vi "Get SMO Port.vi"(8 "error in (no error)":errorcluster, 11 "Inst.FPInstrument in":refnum<class "Inst.FP.lvclass">) -> (0 "error out":errorcluster, 2 "Port":u16, 3 "Inst.FPInstrument out":refnum<class "Inst.FP.lvclass">)   [LabVIEW 2019, in "Inst.FP.lvclass"]
uses:
  Inst.FP.lvclass
  <userlib>/LevyLab/Instrument Framework/Instrument Types/VSource/Instrument.VSource.lvclass
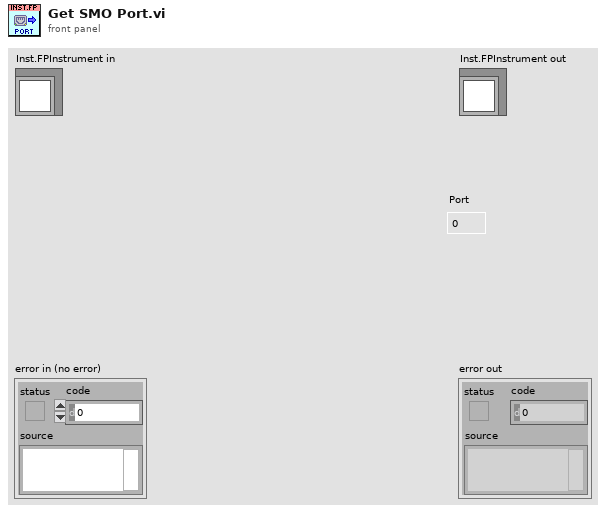
[diagram p1: front panel]
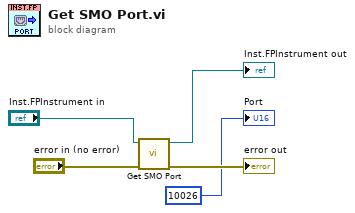
[diagram p0: block diagram]
diagram:
  n1 = call-parent "Get SMO Port.vi"("error in (no error)"="error in (no error)", "Instrument in"="Inst.FPInstrument in") -> ("error out"=→"error out":errorcluster, "Instrument out"=→"Inst.FPInstrument out":refnum<class "Inst.FP.lvclass">)  [unwired: 7 in, 1 out]
  "Port" <- u16 10026 ("Port")
